vi "VisualizeFftResults.vi"() -> ()   [LabVIEW 2018, in "Visualization.lvlib" / "VisualizeAnalysis.lvclass"]
uses:
  VisualizeAnalysis.lvclass
  VisualizeBase/VisualizeBase_class/Requests/VisUserEventType.ctl
  <vilib>/event_ctls.llb/usereventprio.ctl
  Analysis/AnalysisPlugins/FftClass/Typedefs/FftReport.ctl
  <vilib>/Utility/file.llb/Read From Spreadsheet File (DBL).vi
  <vilib>/Utility/error.llb/Error Cluster From Error Code.vi
  <vilib>/ErrorRing/Error Ring.xnode
  VisualizeBase/VisualizeBase_class/VisualizeBase.lvclass
  <userlib>/NIST/NISTErrorLib/NISTErrorLib.lvlib
  Analysis/AnalysisModule/AnalysisModule.lvlib
  Analysis/AnalysisPlugins/FftClass/FFT.lvclass
panel:
  in  "btnReset":bool
  out "DFT":waveform(dbl)[](graph)
  in  "Pause":bool
  in  "btnOpen":bool
  in  "QueName":string="AnalVisQue"
  out "ErrorArray":errorcluster[](array[cluster])
  in  "btnStop":bool
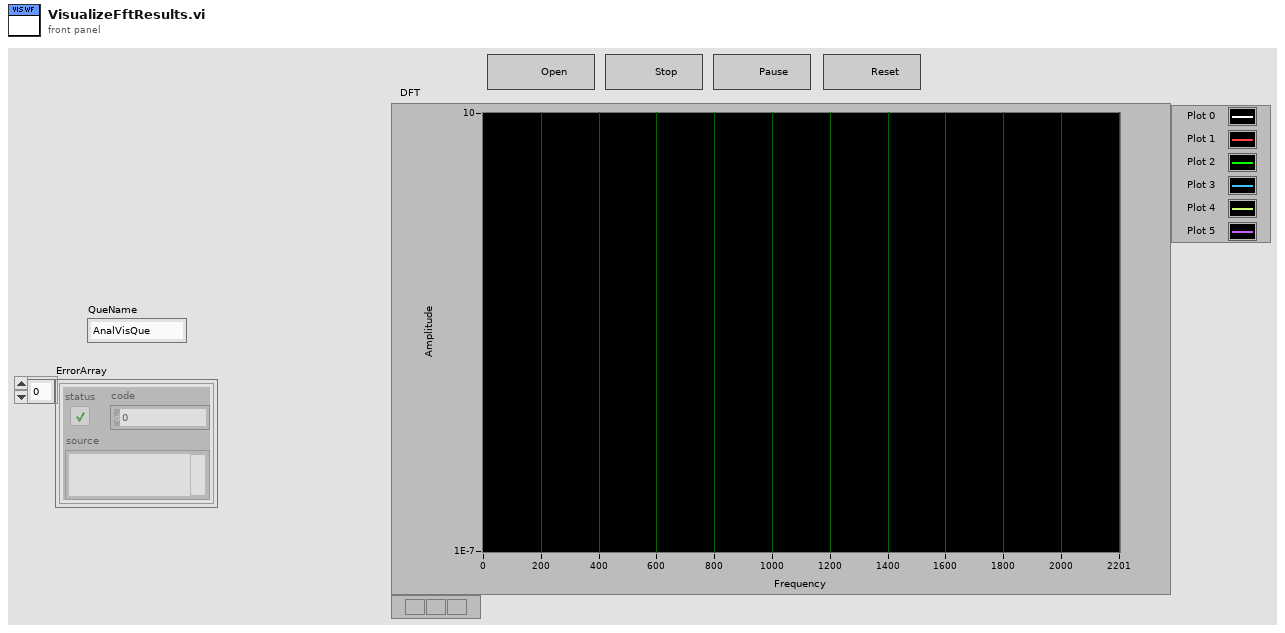
[diagram p1: front panel]
types:
  T1 = typedef "Visualization.lvlib/VisualizeBase.lvclass/VisRequestEvents.ctl" = cluster{"StopRequest":refnum<user-event>, "ResetRequest":refnum<user-event>, "FP Pop In or Out":refnum<user-event>}
  T2 = typedef "AnalysisModule.lvlib/clBroadcastEvents.ctl" = cluster{"DidInit":refnum<user-event>, "StatusUpdate":refnum<user-event>, "ErrorReport":refnum<user-event>, "DidStop":refnum<user-event>, "PathToINI":refnum<user-event>, "Config":refnum<user-event>, "ResultReport":refnum<user-event>, "FunctionClass":refnum<user-event>, "State":refnum<user-event>, "FunctionParams":refnum<user-event>, "Duration":refnum<user-event>}
  T3 = typedef "AnalysisPlugins.lvlib/FFT.lvclass/FftReport.ctl" = cluster{"dF":dbl, "FFT":cdb[][], "F0":dbl}
  T4 = typedef "Visualization.lvlib/VisualizeBase.lvclass/VisUserEventType.ctl" = cluster{"BusIndex":i8, "Data":variant}
  T5 = typedef "usereventprio.ctl" = enum32{"high priority", "normal priority"}
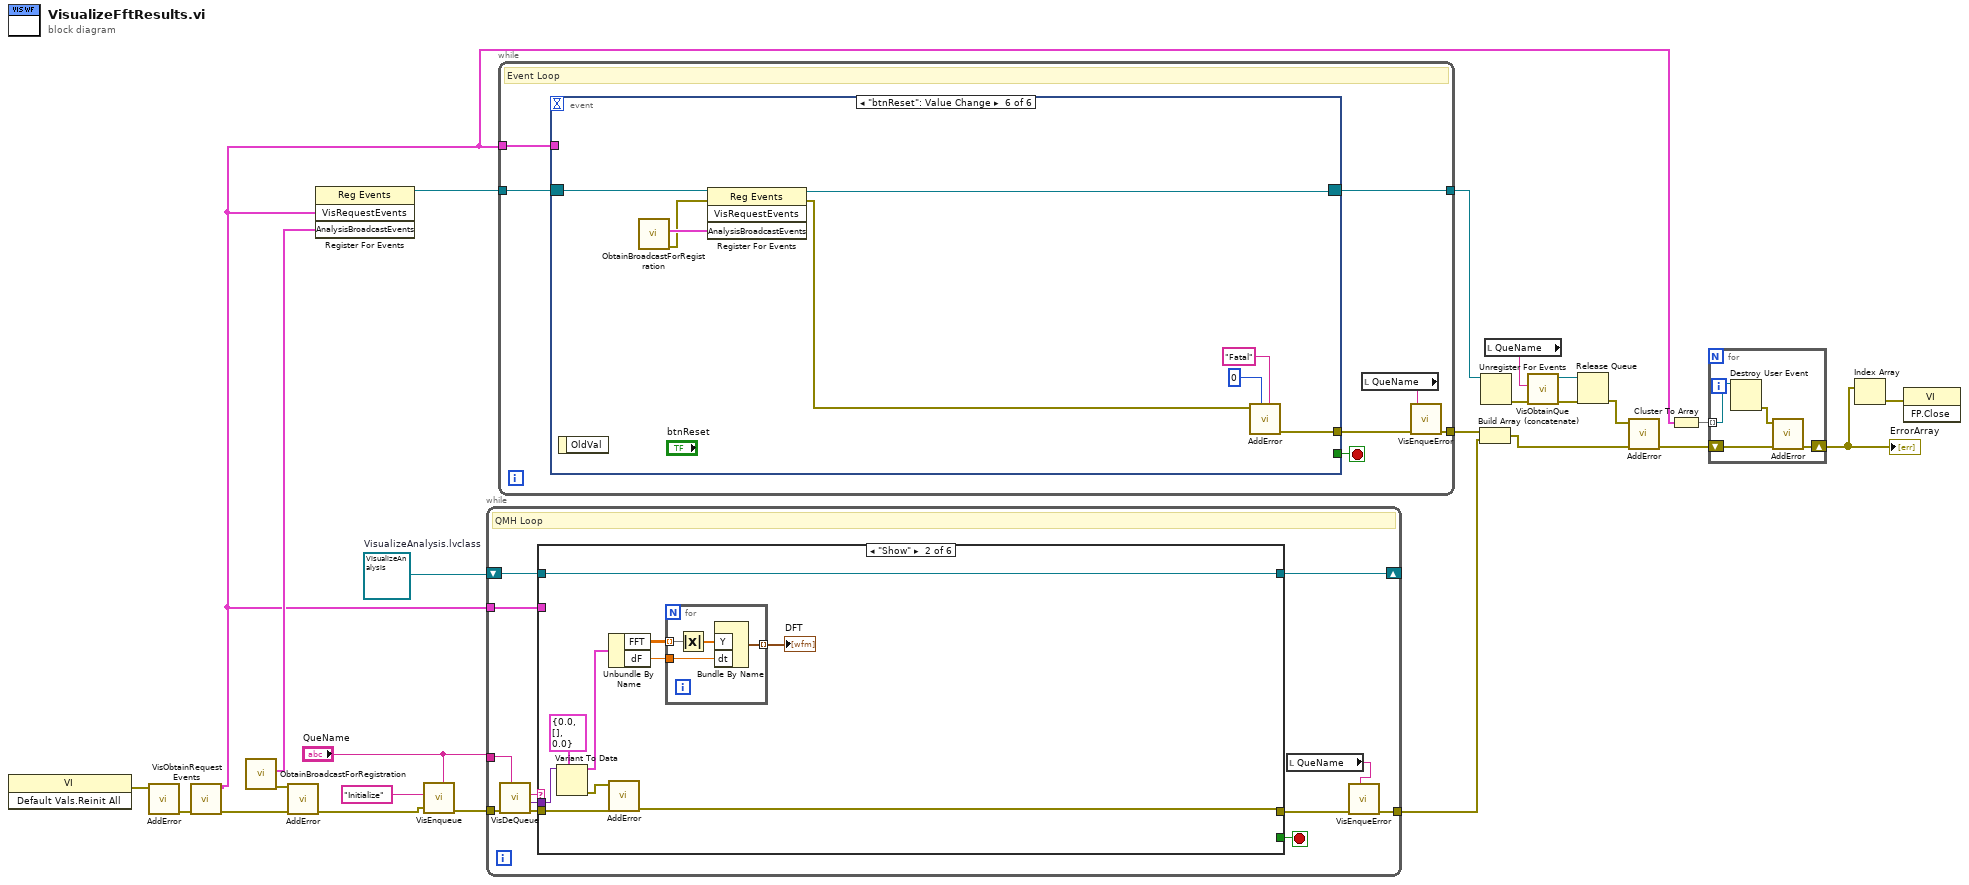
[diagram p0: block diagram]
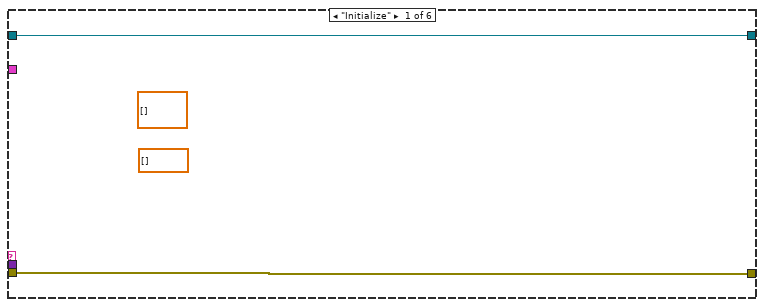
[diagram p2: hidden frame]
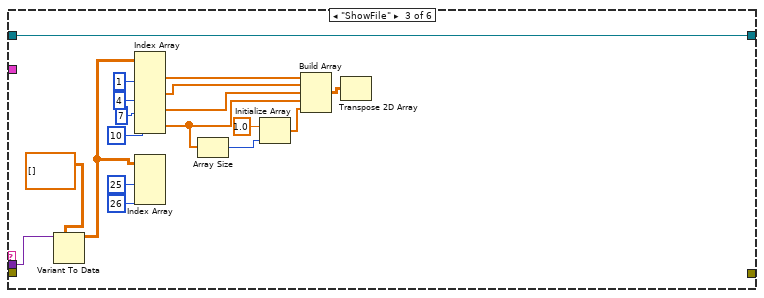
[diagram p3: hidden frame]
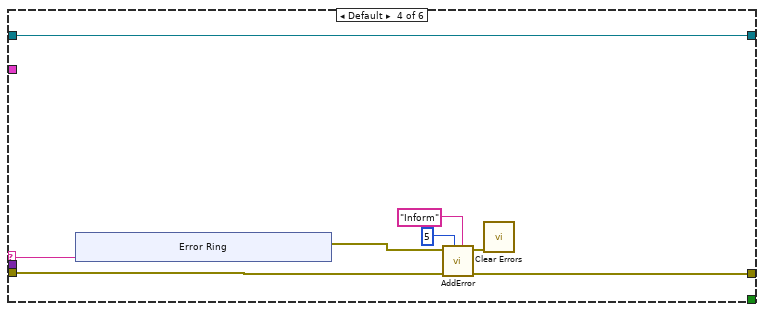
[diagram p4: hidden frame]
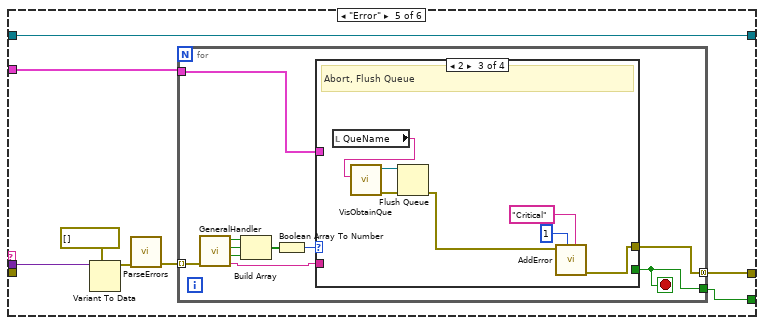
[diagram p5: hidden frame]
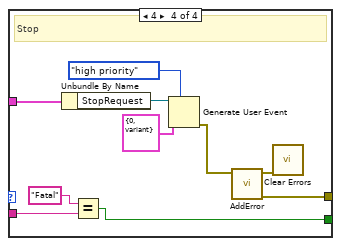
[diagram p8: hidden frame]
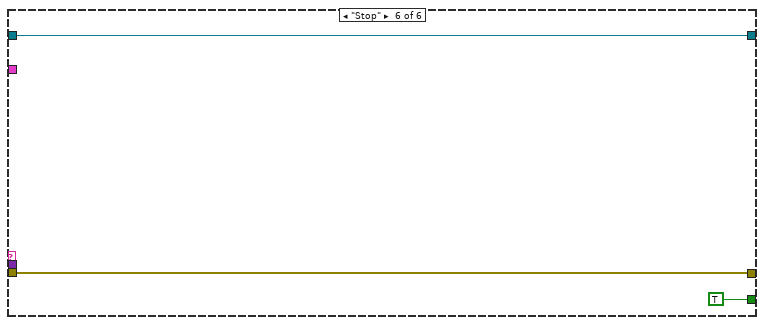
[diagram p9: hidden frame]
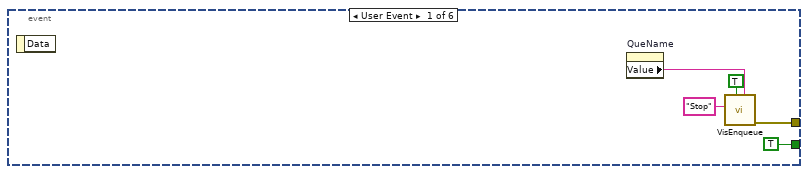
[diagram p10: hidden frame]
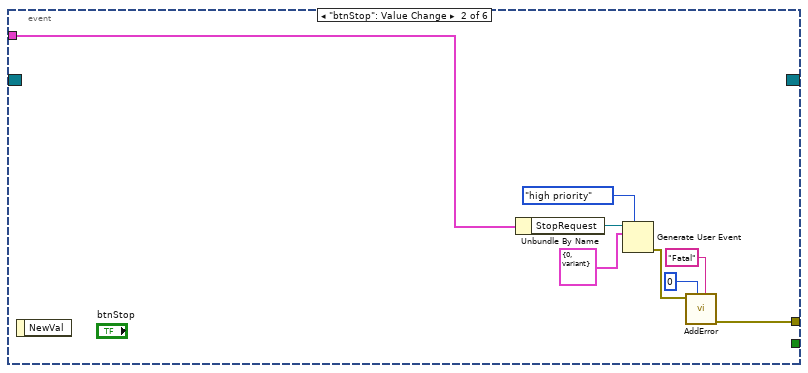
[diagram p11: hidden frame]
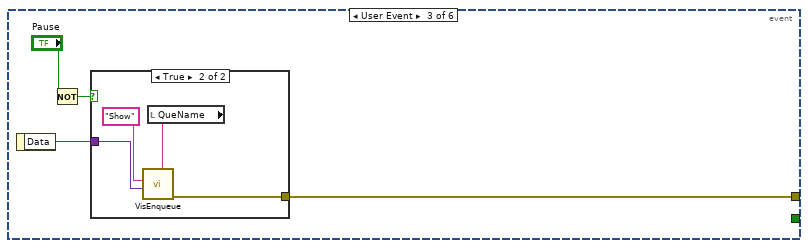
[diagram p12: hidden frame]
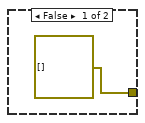
[diagram p13: hidden frame]
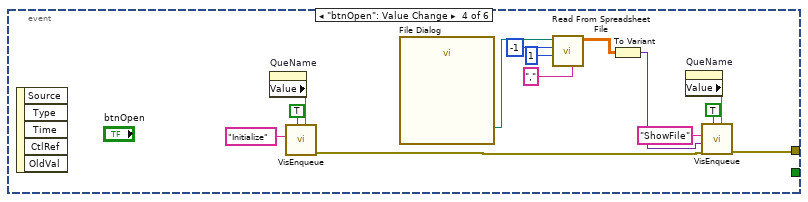
[diagram p14: hidden frame]
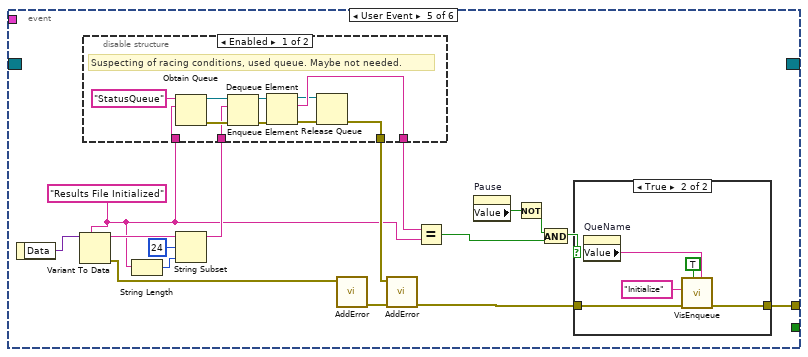
[diagram p15: hidden frame]
diagram:
  w14 = refnum<class "VisualizeAnalysis.lvclass"> refnum  # VisualizeAnalysis.lvclass
  n1 = invoke class="VI" method="Default Vals.Reinit All"() -> (error out=w21:errorcluster)  [unwired: 3 in, 2 out]
  n2 = call <userlib>:"AddError.vi"("error in (no error)"=w21) -> ("ErrorArray Out"=w20:errorcluster[])  [unwired: 9 in, 1 out]
  n3 = call "VisObtainRequestEvents.vi"("Error"=w20) -> ("Error"=w18:errorcluster[], "VisRequestEvents"=w1:T1)  [unwired: 9 in]
  n4 = call "ObtainBroadcastForRegistration.vi"() -> ("error out"=w16:errorcluster, "AnalysisBroadcastEvents"=w19:T2)  [unwired: 10 in]
  n5 = call <userlib>:"AddError.vi"("ErrorArray In"=w18, "error in (no error)"=w16) -> ("ErrorArray Out"=w17:errorcluster[])  [unwired: 8 in, 1 out]
  n6 = register-events(w1, w19) -> (reference out=w13:refnum<event-registration>)  [unwired: 2 in, 1 out]
  n7 = call "VisEnqueue.vi"("QueName"="QueName", "Error"=w17, "Message"="Initialize") -> ("Error"=w24:errorcluster[])  [unwired: 8 in]
  n8 = while {
    tunnel: w24 -> [w37]
    tunnel: [w31] -> w23
    tunnel: "QueName" -> [w29]
    shift-right: [w28] -> _
    shift-left: w14 -> [w27]
    tunnel: w1 -> [w26]
    stop <- w32 stop-if-true
    # "QMH Loop"
    n9 = call "VisDeQueue.vi"("QueName"=w29, "Error"=w37) -> ("Error"=w34:errorcluster[], "Data"=w35:variant, "Message"=w36:string)  [unwired: 7 in]
    n10 = case shown="\"Show\"" w36 {
      selector: w36 -> [_ _ _ w79 _ _]
      tunnel: w35 -> [_ w48 w71 _ w94 _]
      tunnel: w34 -> [w39 w47 _ w77 _ w123]
      tunnel: [w39 w45 _ w76 w90 w123] -> w33
      tunnel: [_ _ _ _ w89 TRUE] -> w32
      tunnel: w27 -> [w38 w49 w69 w72 w88 w122]
      tunnel: [w38 w49 w69 w72 w88 w122] -> w28
      tunnel: w26 -> [_ _ _ _ w87 _]
      frame "Initialize" {
        (unwired) dbl[] [] ("History Data")
        (unwired) dbl[][] [] ("History Data")
      }
      frame "Show" {
        n11 = Variant To Data(type=T3 {"dF"=0.0, "FFT"=[], "F0"=0.0} ("FftReport"), Variant=w48) -> (data=w43:T3, error out=w46:errorcluster)  [unwired: 1 in]
        n12 = Unbundle By Name(w43) -> ("FFT"=w41:cdb[][], "dF"=w42:dbl)
        n13 = call <userlib>:"AddError.vi"("ErrorArray In"=w47, "error in (no error)"=w46) -> ("ErrorArray Out"=w45:errorcluster[])  [unwired: 8 in, 1 out]
        n14 = for {
          tunnel: w42 -> [w53]
          tunnel: w41 -> [w52] mode=indexing
          tunnel: [w50] -> w40 mode=indexing
          n15 = Absolute Value(x=w52) -> (abs(x)=w51:dbl[])
          n16 = Bundle By Name("Y"=w51, "dt"=w53) -> (w50:waveform(dbl))  [unwired: 1 in]
        }
        "DFT" <- w40
      }
      frame "ShowFile" {
        n17 = Variant To Data(type=dbl[][] [], Variant=w71) -> (data=w60:dbl[][])  [unwired: 1 in, 1 out]
        n18 = Index Array(array=w60, index (col) #1=1 ("disabled index (col)"), index (col) #2=4 ("index (col)"), index (col) #3=7 ("index (col)"), index (col) #4=10 ("index (col)")) -> (element #1=w64:dbl[], element #2=w63:dbl[], element #3=w62:dbl[], element #4=w57:dbl[])  [unwired: 4 in]
        n19 = Index Array(array=w60, index (col) #1=25 ("disabled index (col)"), index (col) #2=26 ("index (col)")) -> ()  [unwired: 2 in, 2 out]
        n20 = Array Size(array=w57) -> (size(s)=w56:i32)
        n21 = Initialize Array(1.0 ("element"), w56) -> (w54:dbl[])
        n22 = Build Array(w64, w63, w62, w57, w54) -> (w61:dbl[][])
        n23 = Transpose 2D Array(2D array=w61) -> ()  [unwired: 1 out]
      }
      frame Default {
        n24 = xnode "Error Ring"("parameter 0"=w79) -> ("error out"=w78:errorcluster)
        n25 = call <userlib>:"AddError.vi"("Severity"="Inform" ("String"), "Priority"=u8 5, "ErrorArray In"=w77, "error in (no error)"=w78) -> ("ErrorArray Out"=w76:errorcluster[], "error out"=w75:errorcluster)  [unwired: 6 in]
        n26 = call <vilib>:"Clear Errors.vi"("error in (no error)"=w75) -> ()  [unwired: 5 in, 2 out]
      }
      frame "Error" {
        n27 = Variant To Data(type=errorcluster[] [], Variant=w94) -> (data=w92:errorcluster[])  [unwired: 1 in, 1 out]
        n28 = call <userlib>:"ParseErrors.vi"("ErrorArray"=w92) -> ("ErrorArray"=w91:errorcluster[])  [unwired: 8 in, 2 out]
        n29 = for {
          tunnel: w91 -> [w104] mode=indexing
          tunnel: [w98] -> w90 mode=concatenating
          tunnel: [w96] -> w89
          tunnel: w87 -> [w95]
          stop <- w96 stop-if-true
          n30 = call <userlib>:"GeneralHandler.vi"("error in (no error)"=w104) -> ("Severity"=w97:string, "Stop"=w101:bool, "Abort"=w102:bool, "Continue"=w103:bool)  [unwired: 6 in, 1 out]
          n31 = Build Array(w103, w102, w101) -> (w100:bool[])
          n32 = Boolean Array To Number(Boolean array=w100) -> (number=w99:u32)
          n33 = case shown="2" w99 {
            tunnel: [_ _ w109 w120] -> w98
            tunnel: w97 -> [_ _ _ w115]
            tunnel: [_ _ _ w113] -> w96
            tunnel: w95 -> [_ _ _ w112]
            frame 0, Default {
              # "No Dialog"
            }
            frame 1 {
              # "Continue"
            }
            frame 2 {
              # "Abort, Flush Queue"
              n34 = local read "QueName"() -> (w105:string)
              n35 = call "VisObtainQue.vi"("QueName"=w105) -> ("error out"=w111:errorcluster, "queue out"=w110:refnum<queue>)  [unwired: 9 in]
              n36 = Flush Queue(queue=w110, error in (no error)=w111) -> (error out=w108:errorcluster)  [unwired: 2 out]
              n37 = call <userlib>:"AddError.vi"("Severity"="Critical" ("String"), "Priority"=u8 1, "error in (no error)"=w108) -> ("ErrorArray Out"=w109:errorcluster[])  [unwired: 7 in, 1 out]
            }
            frame 4 {
              # "Stop"
              n38 = Unbundle By Name(w112) -> ("StopRequest"=w121:refnum<user-event>)
              n39 = Equal?(x="Fatal", y=w115) -> (x = y?=w113:bool)
              n40 = Generate User Event(priority (normal)=usereventprio."high priority", user event=w121, event data cluster=T4 {"BusIndex"=0, "Data"=variant} ("event data")) -> (error out=w119:errorcluster)  [unwired: 1 in, 1 out]
              n41 = call <userlib>:"AddError.vi"("error in (no error)"=w119) -> ("ErrorArray Out"=w120:errorcluster[], "error out"=w116:errorcluster)  [unwired: 9 in]
              n42 = call <vilib>:"Clear Errors.vi"("error in (no error)"=w116) -> ()  [unwired: 5 in, 2 out]
            }
          }
        }
      }
      frame "Stop" {
      }
    }
    n43 = local read "QueName"() -> (w30:string)
    n44 = call "VisEnqueError.vi"("QueName"=w30, "Error"=w33) -> ("Error"=w31:errorcluster[])  [unwired: 9 in]
  }
  n45 = while {
    tunnel: [w129] -> w22
    tunnel: w13 -> [w127]
    tunnel: [w126] -> w7
    tunnel: w1 -> [w125]
    stop <- w131 stop-if-true
    # "Event Loop"
    n46 = event shown="[5] \"btnReset\": Value Change" {
      selector: w127 -> [_ _ _ _ _ w209]
      dyn-events: [_ _ _ _ _ w206] -> w126
      timeout: _ -> [_ _ _ _ _ _]
      tunnel: [TRUE _ _ _ _ _] -> w131
      tunnel: [w135 w142 w147 w162 w182 w205] -> w130
      tunnel: w125 -> [_ w137 _ _ _ _]
      event User Event {
        n47 = event-data() -> ()  [unwired: 1 in, 1 out]
        n48 = property on="QueName" class="Str"() -> ("Value"=w132:string)  [unwired: 2 in, 2 out]
        n49 = call "VisEnqueue.vi"("QueName"=w132, "Priority? (F)"=TRUE, "Message"="Stop") -> ("Error"=w135:errorcluster[])  [unwired: 8 in]
      }
      event "btnStop": Value Change {
        n50 = event-data() -> ()  [unwired: 1 in, 1 out]
        n51 = Unbundle By Name(w137) -> ("StopRequest"=w143:refnum<user-event>)
        n52 = Generate User Event(priority (normal)=usereventprio."high priority", user event=w143, event data cluster=T4 {"BusIndex"=0, "Data"=variant} ("event data")) -> (error out=w144:errorcluster)  [unwired: 1 in, 1 out]
        n53 = call <userlib>:"AddError.vi"("Severity"="Fatal" ("String"), "Priority"=u8 0, "error in (no error)"=w144) -> ("ErrorArray Out"=w142:errorcluster[])  [unwired: 7 in, 1 out]
      }
      event User Event {
        n54 = event-data() -> ("Data"=w148:variant)  [unwired: 1 in]
        n55 = Not(x="Pause") -> (.not. x?=w145:bool)
        n56 = case shown="True" w145 {
          tunnel: w148 -> [_ w152]
          tunnel: [errorcluster[] [] ("Error") w151] -> w147
          frame False {
          }
          frame True {
            n57 = local read "QueName"() -> (w153:string)
            n58 = call "VisEnqueue.vi"("QueName"=w153, "Data"=w152, "Message"="Show") -> ("Error"=w151:errorcluster[])  [unwired: 8 in]
          }
        }
      }
      event "btnOpen": Value Change {
        n59 = event-data() -> ()  [unwired: 1 in, 5 out]
        n60 = property on="QueName" class="Str"() -> ("Value"=w159:string)  [unwired: 2 in, 2 out]
        n61 = call "VisEnqueue.vi"("QueName"=w159, "Priority? (F)"=TRUE, "Message"="Initialize") -> ("Error"=w156:errorcluster[])  [unwired: 8 in]
        n62 = call "File Dialog"() -> ("selected path"=w167:path)  [unwired: 12 in, 3 out]
        n63 = call-poly <vilib>:"Read From Spreadsheet File.vi"("delimiter (\\t)"="," ("delimiter (\\t)"), "start of read offset (chars.:0)"=1, "number of rows (all:-1)"=-1, "file path (dialog if empty)"=w167) -> ("all rows"=w161:dbl[][])  [unwired: 3 in, 4 out]
        n64 = To Variant(anything=w161) -> (Variant=w160:variant)
        n65 = property on="QueName" class="Str"() -> ("Value"=w163:string)  [unwired: 2 in, 2 out]
        n66 = call "VisEnqueue.vi"("QueName"=w163, "Priority? (F)"=TRUE, "Error"=w156, "Data"=w160, "Message"="ShowFile") -> ("Error"=w162:errorcluster[])  [unwired: 6 in]
      }
      event User Event {
        w172 = "Results File Initialized" ("Status")
        n67 = event-data() -> ("Data"=w183:variant)  [unwired: 1 in]
        n68 = Variant To Data(type=w172, Variant=w183) -> (data=w180:string, error out=w177:errorcluster)  [unwired: 1 in]
        n69 = String Length(string=w172) -> (length=w173:i32)
        n70 = String Subset(string=w180, offset (0)=24, length (rest)=w173) -> (substring=w175:string)
        n71 = disable-structure shown="Enabled" {
          disable-tunnel: [w187 w195] -> w179
          disable-tunnel: [w184 _] -> w176
          disable-tunnel: w175 -> [w189 w195]
          disable-tunnel: w172 -> [w188 _]
          frame Enabled {
            # "Suspecting of racing conditions, used queue. Maybe not needed."
            n72 = Obtain Queue(name (unnamed)="StatusQueue", element data type=w188) -> (queue out=w193:refnum<queue>, error out=w191:errorcluster)  [unwired: 3 in, 1 out]
            n73 = Enqueue Element(queue=w193, element=w189, error in (no error)=w191) -> (queue out=w192:refnum<queue>, error out=w190:errorcluster)  [unwired: 1 in, 1 out]
            n74 = Dequeue Element(queue=w192, error in (no error)=w190) -> (queue out=w186:refnum<queue>, element=w187:string, error out=w185:errorcluster)  [unwired: 1 in, 1 out]
            n75 = Release Queue(queue=w186, error in (no error)=w185) -> (error out=w184:errorcluster)  [unwired: 1 in, 2 out]
          }
          frame Disabled {
          }
        }
        n76 = call <userlib>:"AddError.vi"("error in (no error)"=w177) -> ("ErrorArray Out"=w178:errorcluster[])  [unwired: 9 in, 1 out]
        n77 = call <userlib>:"AddError.vi"("ErrorArray In"=w178, "error in (no error)"=w176) -> ("ErrorArray Out"=w181:errorcluster[])  [unwired: 8 in, 1 out]
        n78 = Equal?(x=w179, y=w172) -> (x = y?=w170:bool)
        n79 = property on="Pause" class="Bool (strict)"() -> ("Value"=w169:bool)  [unwired: 2 in, 2 out]
        n80 = Not(x=w169) -> (.not. x?=w168:bool)
        n81 = And(x=w168, y=w170) -> (x .and. y?=w171:bool)
        n82 = case shown="True" w171 {
          tunnel: [w196 w198] -> w182
          tunnel: w181 -> [w196 w197]
          frame False {
          }
          frame True {
            n83 = property on="QueName" class="Str"() -> ("Value"=w199:string)  [unwired: 2 in, 2 out]
            n84 = call "VisEnqueue.vi"("QueName"=w199, "Priority? (F)"=TRUE, "Error"=w197, "Message"="Initialize") -> ("Error"=w198:errorcluster[])  [unwired: 7 in]
          }
        }
      }
      event "btnReset": Value Change {
        n85 = event-data() -> ()  [unwired: 1 in, 1 out]
        n86 = call "ObtainBroadcastForRegistration.vi"() -> ("error out"=w207:errorcluster, "AnalysisBroadcastEvents"=w208:T2)  [unwired: 10 in]
        n87 = register-events(reference=w209, error in=w207, w208) -> (reference out=w206:refnum<event-registration>, error out=w204:errorcluster)  [unwired: 1 in]
        n88 = call <userlib>:"AddError.vi"("Severity"="Fatal", "Priority"=u8 0, "error in (no error)"=w204) -> ("ErrorArray Out"=w205:errorcluster[])  [unwired: 7 in, 1 out]
      }
    }
    n89 = local read "QueName"() -> (w128:string)
    n90 = call "VisEnqueError.vi"("QueName"=w128, "Error"=w130) -> ("Error"=w129:errorcluster[])  [unwired: 9 in]
  }
  n91 = Build Array (concatenate)(w22, w23) -> (w6:errorcluster[])
  n92 = Unregister For Events(event registration refnum=w7) -> (error out=w9:errorcluster)  [unwired: 1 in]
  n93 = local read "QueName"() -> (w3:string)
  n94 = call "VisObtainQue.vi"("error in (no error)"=w9, "QueName"=w3) -> ("error out"=w10:errorcluster, "queue out"=w11:refnum<queue>)  [unwired: 8 in]
  n95 = Release Queue(queue=w11, error in (no error)=w10) -> (error out=w12:errorcluster)  [unwired: 1 in, 2 out]
  n96 = call <userlib>:"AddError.vi"("ErrorArray In"=w6, "error in (no error)"=w12) -> ("ErrorArray Out"=w2:errorcluster[])  [unwired: 8 in, 1 out]
  n97 = Cluster To Array(cluster=w1) -> (array=w8:refnum<user-event>[])
  n98 = for {
    tunnel: w8 -> [w213] mode=indexing
    shift-right: [w212] -> w5
    shift-left: w2 -> [w211]
    n99 = Destroy User Event(user event=w213) -> (error out=w210:errorcluster)  [unwired: 1 in]
    n100 = call <userlib>:"AddError.vi"("ErrorArray In"=w211, "error in (no error)"=w210) -> ("ErrorArray Out"=w212:errorcluster[])  [unwired: 8 in, 1 out]
  }
  "ErrorArray" <- w5
  n101 = Index Array(array=w5) -> (element=w4:errorcluster)  [unwired: 1 in]
  n102 = invoke class="VI" method="FP.Close"(error in=w4) -> ()  [unwired: 2 in, 3 out]
